vi "Run.vi"(8 "Column":i32, 9 "Row":i32, 10 "Maze (0: Empty, -1: Enemy. 1: Teammate)":i32[](array[numeric]), 11 "Runner in":refnum<class "Rain.lvclass">) -> (0 "Replicated":refnum<class "Square.lvclass">, 1 "Direction":T2, 2 "Action":T3, 3 "Runner out":refnum<class "Rain.lvclass">)   [LabVIEW 2015, in "Rain.lvclass"]
uses:
  Rain.lvclass
  Type Defs/Action Enum.ctl
  Type Defs/Direction Enum.ctl
  Square/Square.lvclass
  Carl/Formics/Attack Options.ctl
  SubVIs/Read-Only Globals.vi
  Carl/Common/Reverse Direction.vi
  Carl/Common/Common.lvlib
  Type Defs/SB Type Defs.lvlib
  Carl/Formics/Formics.lvclass
panel:
  in  "Attack":T1
  # "NW\nN\nNE\nE\nSE\nS\nSW\nW"
  # "NOTICE - YOU MUST NOT REMOVE THIS NOTICE. PER THE FOLLOWING LICENSE, YOU MAY REPRODUCE THIS SOFTWARE PROVIDED YOU FOLLOW THE TERMS\nOF THE LICENSE.\n\n---BEGIN BSD LICENSE (http://opensource.org/licenses/BSD-2-Clause)---\nCopyright (c) 2015, Endigit, Inc. <robert@endigit.com>\nAll rights reserved.\n\nRedistribution and use in source and binary forms, with or without modification, are permitted provided that the following conditions are met:\n\n1. Redistributions of source code must retain the above copyright notice, this list of conditions and the following disclaimer.\n\n2. Redistributions in binary form must reproduce the above copyright notice, this list of conditions and the following disclaimer in the documentation and/or other \nmaterials provided with the distribution.\n\nTHIS SOFTWARE IS PROVIDED BY THE COPYRIGHT HOLDERS AND CONTRIBUTORS \"AS IS\" AND ANY EXPRESS OR IMPLIED WARRANTIES, INCLUDING, BUT NOT \nLIMITED TO, THE IMPLIED WARRANTIES OF MERCHANTABILITY AND FITNESS FOR A PARTICULAR PURPOSE ARE DISCLAIMED. IN NO EVENT SHALL THE COPYRIGHT \nHOLDER OR CONTRIBUTORS BE LIABLE FOR ANY DIRECT, INDIRECT, INCIDENTAL, SPECIAL, EXEMPLARY, OR CONSEQUENTIAL DAMAGES (INCLUDING, BUT NOT \nLIMITED TO, PROCUREMENT OF SUBSTITUTE GOODS OR SERVICES; LOSS OF USE, DATA, OR PROFITS; OR BUSINESS INTERRUPTION) HOWEVER CAUSED AND ON \nANY THEORY OF LIABILITY, WHETHER IN CONTRACT, STRICT LIABILITY, OR TORT (INCLUDING NEGLIGENCE OR OTHERWISE) ARISING IN ANY WAY OUT OF THE USE \nOF THIS SOFTWARE, EVEN IF ADVISED OF THE POSSIBILITY OF SUCH DAMAGE.\n---END BSD LICENSE---"
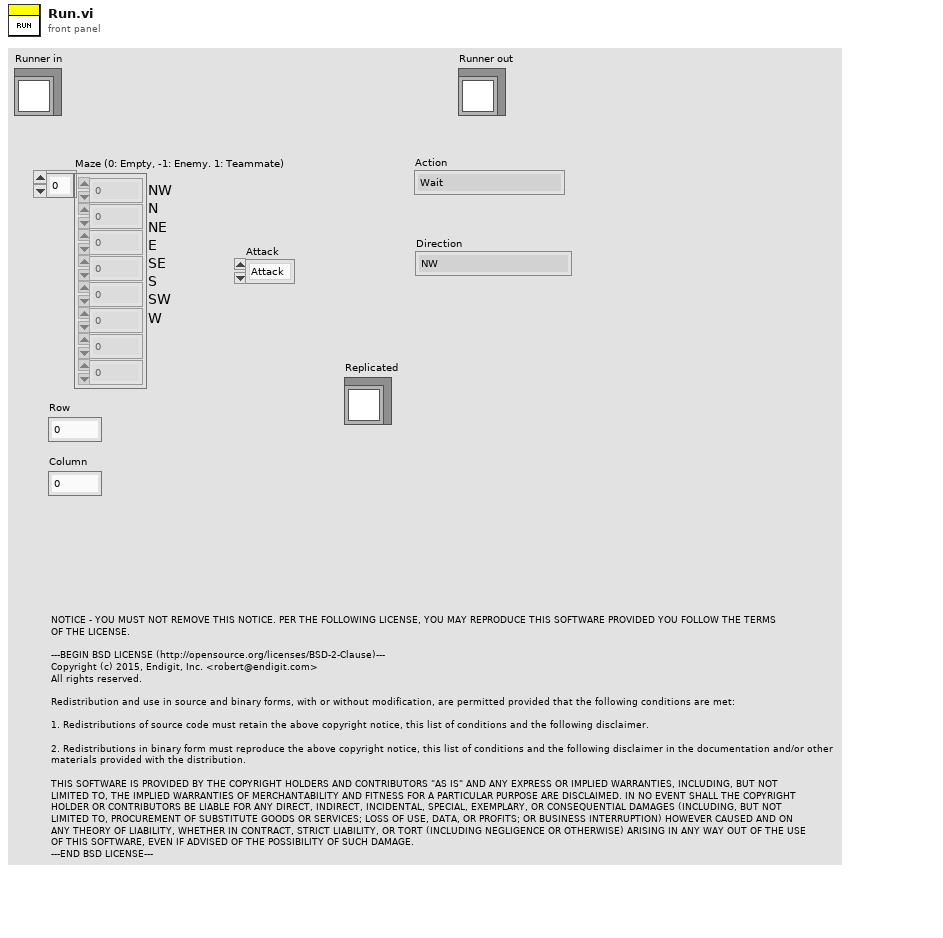
[diagram p1: front panel]
types:
  T1 = typedef "Formics.lvclass/Attack Options.ctl" = enum16{"Attack", "Run", "Distract"}
  T2 = typedef "SB Type Defs.lvlib/Direction Enum.ctl" = enum16{"NW", "N", "NE", "E", "SE", "S", "SW", "W"}
  T3 = typedef "SB Type Defs.lvlib/Action Enum.ctl" = enum16{"Wait", "Move", "Attack", "Replicate"}
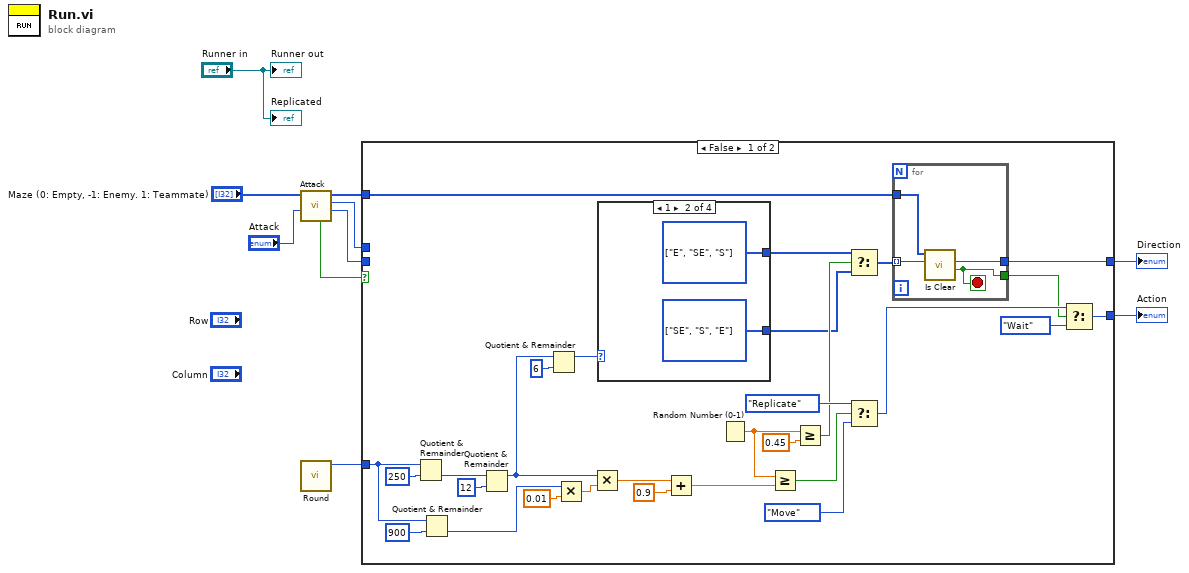
[diagram p0: block diagram]
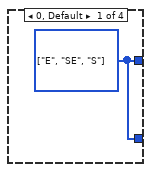
[diagram p2: hidden frame]
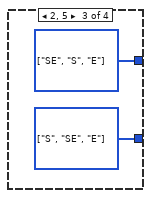
[diagram p3: hidden frame]
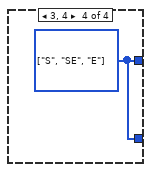
[diagram p4: hidden frame]
diagram:
  n1 = call "Attack.vi"("Attack?"="Attack", "Maze (0: Empty, -1: Enemy. >0: Teammate"="Maze (0: Empty, -1: Enemy. 1: Teammate)") -> ("Direction"=w9:i32, "Action"=w7:T3, "Maze (0: Empty, -1: Enemy. >0: Teammate 2"=w5:i32[], "Enemy Found?"=w10:bool)  [unwired: 4 in, 2 out]
  n2 = call "Round.vi"() -> ("Round"=w2:i32)  [unwired: 11 in]
  n3 = case shown="False" w10 {
    tunnel: w9 -> [_ w51]
    tunnel: [w32 w51] -> w8
    tunnel: w7 -> [_ w50]
    tunnel: [w36 w50] -> w6
    tunnel: w5 -> [w33 _]
    tunnel: w2 -> [w15 _]
    frame False {
      n4 = Quotient & Remainder(x=w15, y=250) -> (floor(x/y)=w23:i32)  [unwired: 1 out]
      n5 = Quotient & Remainder(x=w15, y=900) -> (floor(x/y)=w13:i32)  [unwired: 1 out]
      n6 = Quotient & Remainder(x=w23, y=12) -> (x-y*floor(x/y)=w17:i32)  [unwired: 1 out]
      n7 = Quotient & Remainder(x=w17, y=6) -> (x-y*floor(x/y)=w16:i32)  [unwired: 1 out]
      n8 = Multiply(x=w13, y=0.01) -> (x*y=w11:dbl)
      n9 = Multiply(x=w17, y=w11) -> (x*y=w22:dbl)
      n10 = case shown="1" w16 {
        tunnel: [w40 w42 w44 w45] -> w27
        tunnel: [w40 w41 w43 w45] -> w28
        frame 0, Default {
          w40 = T2[] [enum."E", enum."SE", enum."S"] items=["NW", "N", "NE", "E", "SE", "S", "SW", "W"]
        }
        frame 1 {
          w41 = T2[] [enum."SE", enum."S", enum."E"] items=["NW", "N", "NE", "E", "SE", "S", "SW", "W"]
          w42 = T2[] [enum."E", enum."SE", enum."S"] items=["NW", "N", "NE", "E", "SE", "S", "SW", "W"]
        }
        frame 2, 5 {
          w43 = T2[] [enum."S", enum."SE", enum."E"] items=["NW", "N", "NE", "E", "SE", "S", "SW", "W"]
          w44 = T2[] [enum."SE", enum."S", enum."E"] items=["NW", "N", "NE", "E", "SE", "S", "SW", "W"]
        }
        frame 3, 4 {
          w45 = T2[] [enum."S", enum."SE", enum."E"] items=["NW", "N", "NE", "E", "SE", "S", "SW", "W"]
        }
      }
      n11 = Add(x=w22, y=0.9) -> (x+y=w20:dbl)
      n12 = Random Number (0-1)() -> (number: 0 to 1=w25:dbl)
      n13 = Greater Or Equal?(x=w25, y=w20) -> (x >= y?=w31:bool)
      n14 = Greater Or Equal?(x=w25, y=0.45) -> (x >= y?=w29:bool)
      n15 = Select(t=w27, s=w29, f=w28) -> (s? t:f=w26:T2[])
      n16 = Select(t=Action_Enum."Replicate" ("Action"), s=w31, f=Action_Enum."Move" ("Action")) -> (s? t:f=w37:T3)
      n17 = for {
        tunnel: [w47] -> w35
        tunnel: w26 -> [w49] mode=indexing
        tunnel: w33 -> [w48]
        tunnel: [w46] -> w32
        stop <- w47 stop-if-true
        n18 = call "Is Clear.vi"("Direction"=w49, "Maze"=w48) -> ("Can Move?"=w47:bool, "Direction Out"=w46:T2)  [unwired: 7 in, 1 out]
      }
      n19 = Select(t=w37, s=w35, f=Action_Enum."Wait" ("Action")) -> (s? t:f=w36:T3)
    }
    frame True {
    }
  }
  "Action" <- w6
  "Direction" <- w8
  "Runner out" <- "Runner in"
  "Replicated" <- "Runner in"
